vi "FPGA.vi"() -> ()   [LabVIEW 2013]
uses:
  <vilib>/Platform/TimedLoop/XDataNode/timing_clust.ctl
  <vilib>/Platform/TimedLoop/XDataNode/nitl_modes.ctl
  <vilib>/Platform/TimedLoop/XDataNode/wakeup.ctl
  <vilib>/rvi/Emulation/niFpgaSctlEmulationGetInTimedLoop.vi
  <vilib>/rvi/Emulation/niFpgaEmulationReportErrorSimple.vi
  <vilib>/rvi/Emulation/niFpgaGetClockAttributes.vi
  <vilib>/rvi/Emulation/niFpgaCriticalErrorInLSC.vi
  <vilib>/rvi/eio/common/nirviEmuTemplateMethod_errors.vi
  <vilib>/rvi/DataTransferAndStorage/Container/Common/niFpgaContainerExecOnDevCompGetState.vi
  <vilib>/rvi/FIFO/Fifo_Resource/nirvififoEmulationWriteFpgaImpl.vi
  <vilib>/rvi/DataTransferAndStorage/Container/Common/niFpgaContainerGetUniqueNameForEmu.vi
  <vilib>/rvi/interface/RandomDataEmulation/nirviRandomDataFPGAFIFO.vi
  <vilib>/rvi/interface/RandomDataEmulation/niFpgaRandomDataHandleErrors.vi
  <vilib>/rvi/eio/common/nirviEmuReportErrorAndStop.vi
  <vilib>/Platform/TimedLoop/XDataNode/XDataNode.xnode
  <vilib>/eio/EIONode/EIONode.xnode
  <vilib>/rvi/DataTransferAndStorage/Container/XNode/niFpgaContainer.xnode
  <vilib>/rvi/FIFO/Fifo_Resource/niFpgaFifoEmulationRefIn.vi
  <vilib>/Platform/TimedLoop/XDataNode/XDNodeRunTimeDep.lvlib
panel:
  in  "FIFO In 2":refnum<k21>="FIFO"
  in  "Boolean":bool
  out "FIFO Out":refnum<k21>
  in  "FIFO In":refnum<k21>="FIFO"
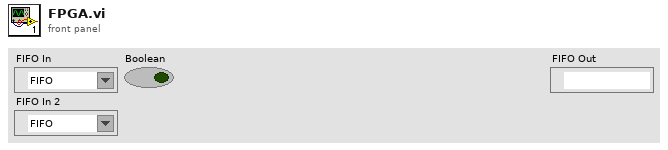
[diagram p1: front panel]
types:
  T1 = typedef "XDNodeRunTimeDep.lvlib/timing_clust.ctl" = cluster{"Expected End [f-1]":u64, "Actual End [f-1]":u64, "Finished Late? [f-1]":bool, "Expected End [i-1]":u64, "Actual End [i-1]":u64, "Finished Late? [i-1]":bool, "Expected Start [i]":u64, "Actual Start [i]":u64, "Expected Start [f]":u64, "Actual Start [f]":u64, "Source Name":string, "Structure Name":string, "Period":i64, "Deadline":i64, "Offset":i64, "Start":i64, "Priority":i32, "Timeout":i32, "Mode":T2, "Wakeup Reason":T3, "Error":errorcluster, "Source Type":string, "Secondary Source Type":string, "Global End Time":u64, "Global Start Time":u64, "Frame Duration":u64, "Iteration Duration":u64, "Assigned CPU":i32, "I/O Scan Engine Mode":u32}
  T2 = typedef "XDNodeRunTimeDep.lvlib/nitl_modes.ctl" = enum32{"No Change", "Process missed periods, maintain original phase", "Discard missed periods, maintain original phase", "Process missed periods, ignore original phase", "Discard missed periods, ignore original phase"}
  T3 = typedef "XDNodeRunTimeDep.lvlib/wakeup.ctl" = enum32{"Normal", "Aborted", "Asynchronous wakeup", "Timing source error", "Timed loop error", "Timeout"}
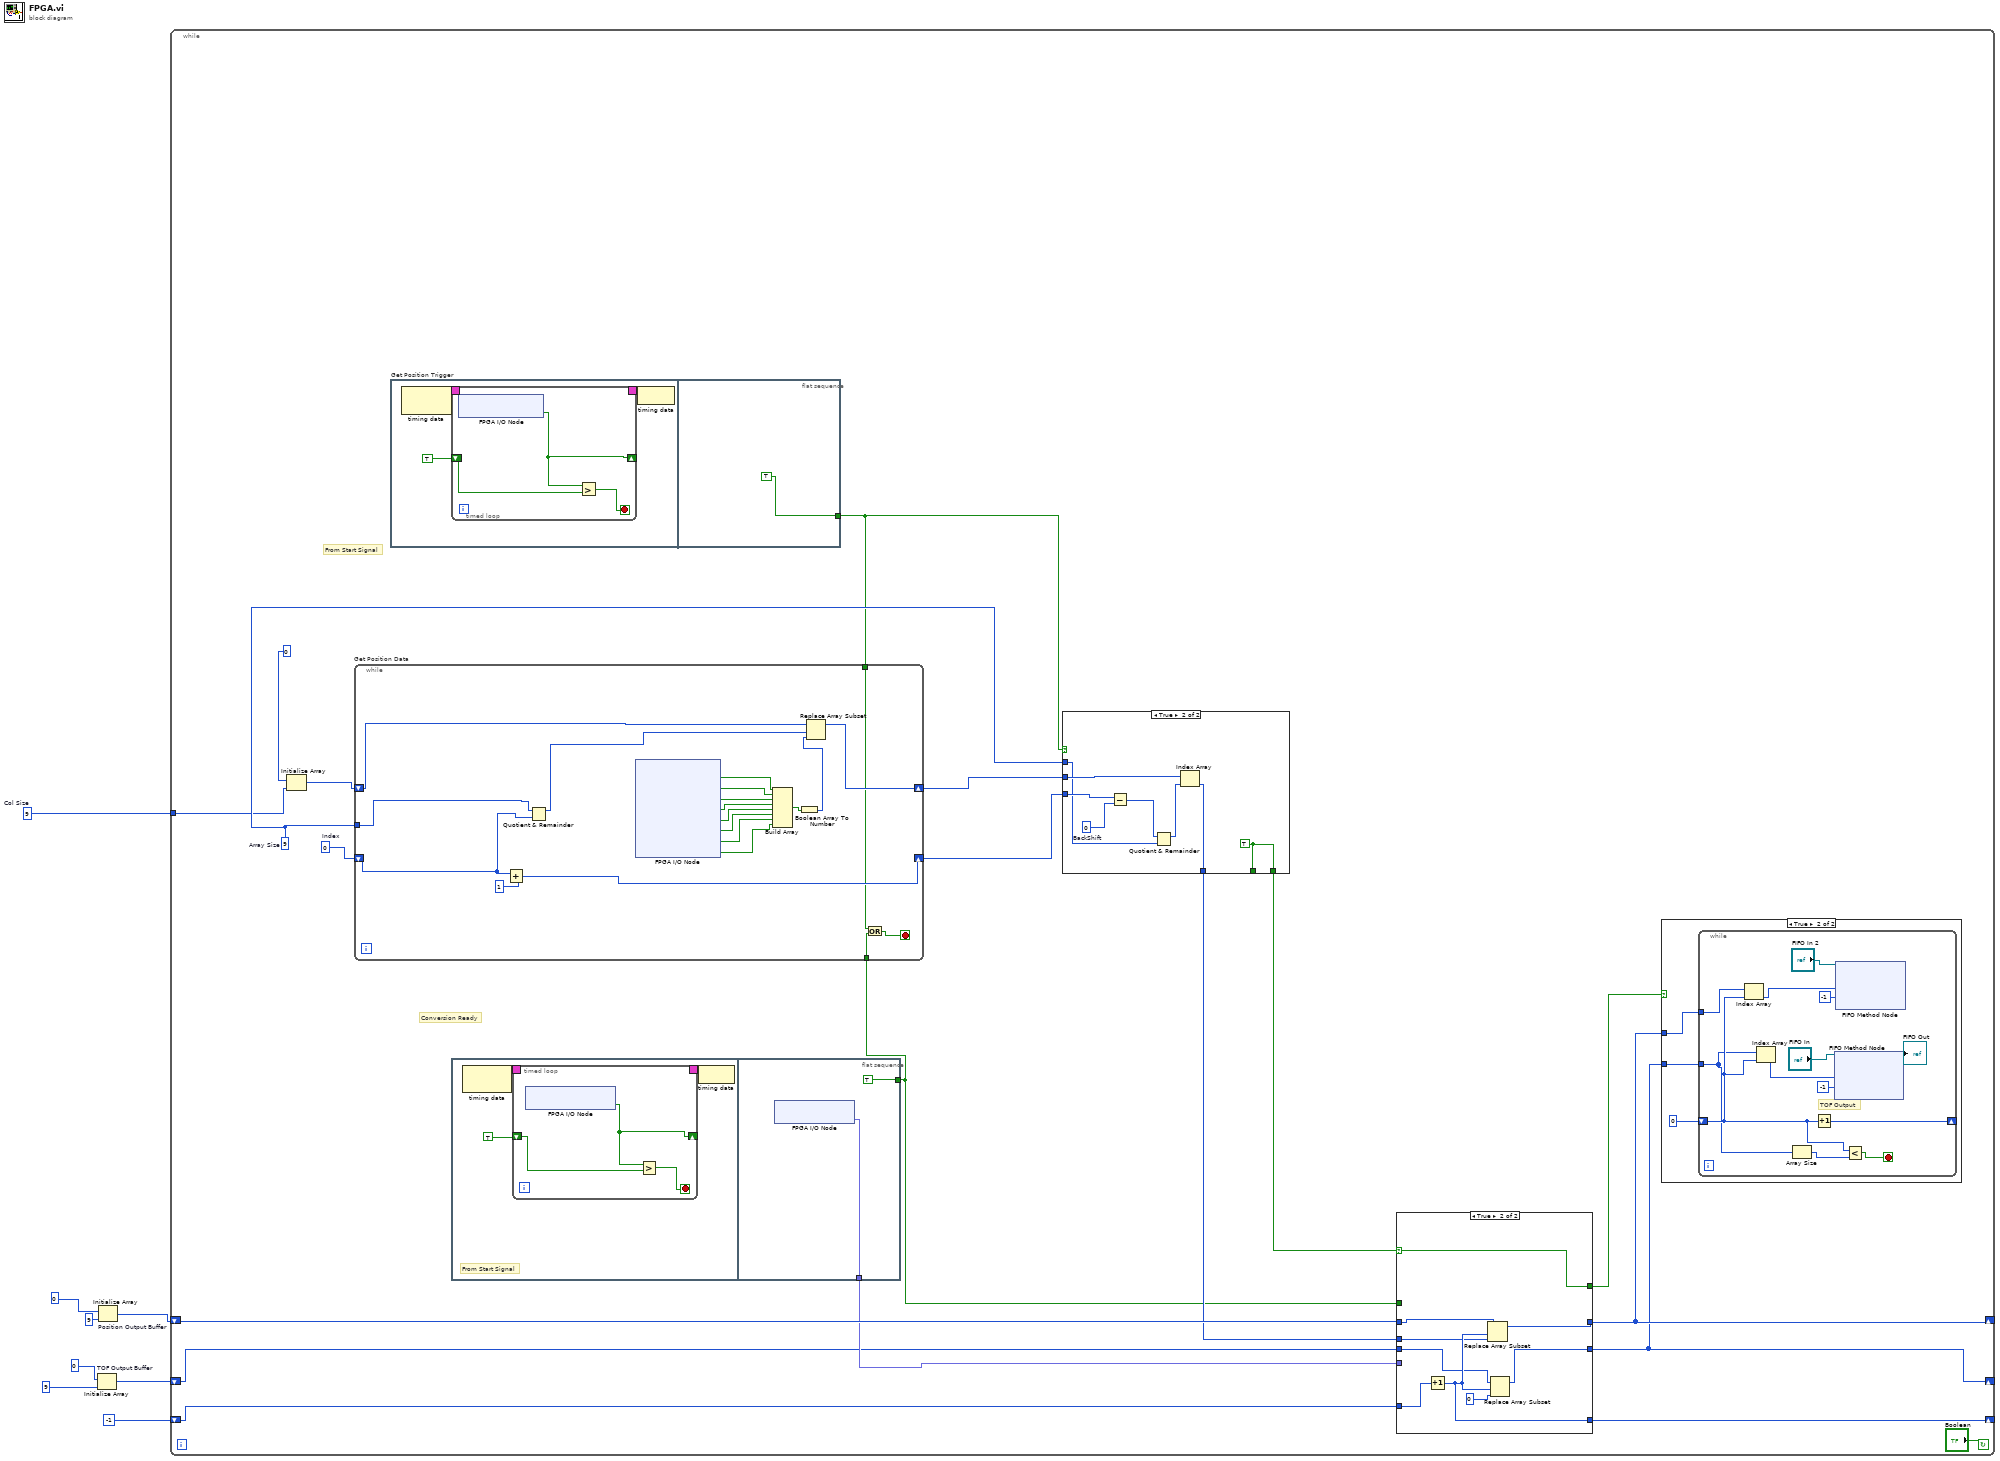
[diagram p0: block diagram]
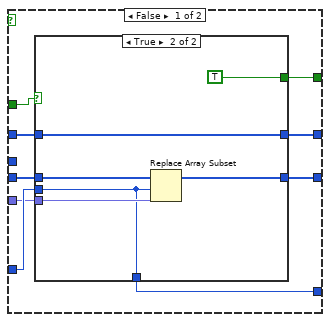
[diagram p2: hidden frame]
diagram:
  w6 = 9  # Col Size
  n1 = Initialize Array "TOF Output Buffer"(i16 0, i16 9) -> (w1:i16[])
  n2 = Initialize Array "Position Output Buffer"(i16 0, 9 ("dimension size")) -> (w5:i16[])
  n3 = while {
    tunnel: w6 -> [w14]
    shift-right: [w20] -> _
    shift-left: w5 -> [w22]
    shift-right: [w18] -> _
    shift-left: -1 -> [w19]
    shift-right: [w12] -> _
    shift-left: w1 -> [w13]
    stop <- "Boolean" continue-if-true
    w23 = i16 9  # Array Size
    w28 = i16 0  # Index
    # "Conversion Ready"
    # "From Start Signal"
    n4 = Initialize Array(i16 0, w14) -> (w26:i16[])
    n5 = while "Get Position Data" {
      shift-right: [w39] -> w24
      shift-left: w28 -> [w30]
      tunnel: w23 -> [w31]
      shift-right: [w38] -> w25
      shift-left: w26 -> [w37]
      tunnel: w11 -> [w33]
      tunnel: w9 -> [w32]
      stop <- w34 stop-if-true
      n6 = Add(x=w30, y=i16 1) -> (x+y=w39:i16)
      n7 = Quotient & Remainder(x=w31, y=w30) -> (x-y*floor(x/y)=w29:i16)  [unwired: 1 out]
      n8 = xnode "FPGA I/O Node"() -> ("Connector0/DIO1"=w48:bool, "Connector0/DIO2"=w47:bool, "Connector0/DIO3"=w46:bool, "Connector0/DIO4"=w45:bool, "Connector0/DIO5"=w44:bool, "Connector0/DIO6"=w43:bool, "Connector0/DIO7"=w42:bool, "Connector0/DIO8"=w41:bool)  [unwired: 8 in, 8 out]
      n9 = Build Array(w48, w47, w46, w45, w44, w43, w42, w41) -> (w36:bool[])
      n10 = Boolean Array To Number(Boolean array=w36) -> (number=w35:u8)
      n11 = Replace Array Subset(array=w37, new element=w35, index=w29) -> (w38:i16[])
      n12 = Or(x=w32, y=w33) -> (x .or. y?=w34:bool)
    }
    n13 = flat-sequence "Get Position Trigger" {
      tunnel: [TRUE] -> w9
      frame #0 {
        n14 = node-c288() -> (w111:T1)  [unwired: 1 in]
        n15 = timed-loop {
          timing: w111 -> [_]
          timing-out: [_] -> w110
          shift-right: [w112] -> _
          shift-left: TRUE ("Connector0/DIO0") -> [w113]
          stop <- w114 stop-if-true
          n16 = xnode "FPGA I/O Node"() -> ("Connector0/DIO0"=w112:bool)  [unwired: 1 in, 1 out]
          n17 = Greater?(x=w112, y=w113) -> (0:w114:bool)
        }
        n18 = node-c288(w110) -> ()
      }
      frame #1 {
      }
    }
    n19 = flat-sequence {
      tunnel: [TRUE] -> w11
      tunnel: [w99] -> w17
      frame #0 {
        # "From Start Signal"
        n20 = node-c288() -> (w91:T1)  [unwired: 1 in]
        n21 = timed-loop {
          timing: w91 -> [_]
          timing-out: [_] -> w90
          shift-right: [w92] -> _
          shift-left: TRUE ("Connector0/DIO0") -> [w93]
          stop <- w94 stop-if-true
          n22 = xnode "FPGA I/O Node"() -> ("Connector0/DIO31"=w92:bool)  [unwired: 1 in, 1 out]
          n23 = Greater?(x=w92, y=w93) -> (0:w94:bool)
        }
        n24 = node-c288(w90) -> ()
      }
      frame #1 {
        n25 = xnode "FPGA I/O Node"() -> ("Connector1/AI0"=w99:fxp<+/-,27,5>)  [unwired: 1 in, 1 out]
      }
    }
    n26 = case shown="True" w9 {
      tunnel: w25 -> [_ w108]
      tunnel: w24 -> [_ w107]
      tunnel: w23 -> [_ w105]
      tunnel: [_ w103] -> w16
      tunnel: [_ w101] -> w10
      tunnel: [_ w101] -> _
      frame False {
      }
      frame True {
        w101 = TRUE
        w106 = i16 0  # BackShift
        n27 = Subtract(x=w107, y=w106) -> (x-y=w104:i16)
        n28 = Quotient & Remainder(x=w104, y=w105) -> (x-y*floor(x/y)=w102:i16)  [unwired: 1 out]
        n29 = Index Array(array=w108, index=w102) -> (element=w103:i16)
      }
    }
    n30 = case shown="True" w10 {
      selector: w10 -> [_ w64]
      tunnel: w22 -> [w57 w65]
      tunnel: [w56 w72] -> w20
      tunnel: w11 -> [w55 _]
      tunnel: [w54 w64] -> w21
      tunnel: w19 -> [w52 w71]
      tunnel: [w49 w70] -> w18
      tunnel: w13 -> [w53 w67]
      tunnel: [w50 w69] -> w12
      tunnel: w17 -> [w51 _]
      tunnel: w16 -> [_ w66]
      frame False {
        n31 = case shown="True" w55 {
          tunnel: w57 -> [_ w62]
          tunnel: [_ w62] -> w56
          tunnel: [_ TRUE] -> w54
          tunnel: w53 -> [_ w59]
          tunnel: w52 -> [_ w58]
          tunnel: [_ w61] -> w50
          tunnel: w51 -> [_ w60]
          tunnel: [_ w58] -> w49
          frame False {
          }
          frame True {
            n32 = Replace Array Subset(array=w59, new element=w60, index=w58) -> (w61:i16[])
          }
        }
      }
      frame True {
        n33 = Increment(x=w71) -> (x+1=w70:i32)
        n34 = Replace Array Subset(array=w65, new element=w66, index=w70) -> (w72:i16[])
        n35 = Replace Array Subset(array=w67, new element=0, index=w70) -> (w69:i16[])
      }
    }
    n36 = case shown="True" w21 {
      tunnel: w20 -> [_ w73]
      tunnel: w12 -> [_ w74]
      frame False {
      }
      frame True {
        n37 = while {
          shift-right: [w87] -> _
          shift-left: 0 -> [w86]
          tunnel: w74 -> [w77]
          tunnel: w73 -> [w88]
          stop <- w84 stop-if-true
          # "TOF Output"
          n38 = Index Array(array=w88, index=w86) -> (element=w78:i16)
          n39 = Index Array(array=w77, index=w86) -> (element=w80:i16)
          n40 = Array Size(array=w77) -> (size(s)=w85:i32)
          n41 = Increment(x=w86) -> (x+1=w87:i32)
          n42 = xnode ("FIFO Method Node")("Element"=w80, "Timeout"=-1, "FIFO In"="FIFO In") -> ("FIFO Out"=→"FIFO Out":refnum<k21>)  [unwired: 1 out]
          n43 = xnode ("FIFO Method Node")("Element"=w78, "Timeout"=-1, "FIFO In"="FIFO In 2") -> ()  [unwired: 2 out]
          n44 = Less?(x=w86, y=w85) -> (x < y?=w84:bool)
        }
      }
    }
  }
